vi "Write Priority.vi"(8 "error in (no error)":errorcluster, 10 "Priority":u8, 11 "SearchPriority in":refnum<class "SearchPriority.lvclass">) -> (0 "error out":errorcluster, 3 "SearchPriority out":refnum<class "SearchPriority.lvclass">)   [LabVIEW 2009, in "SearchPriority.lvclass"]
uses:
  SearchPriority.lvclass
  SearchPriority.lvclass/SearchPriority.ctl
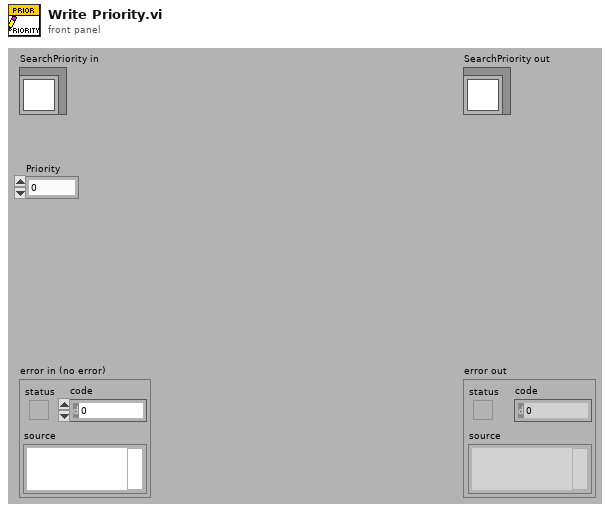
[diagram p1: front panel]
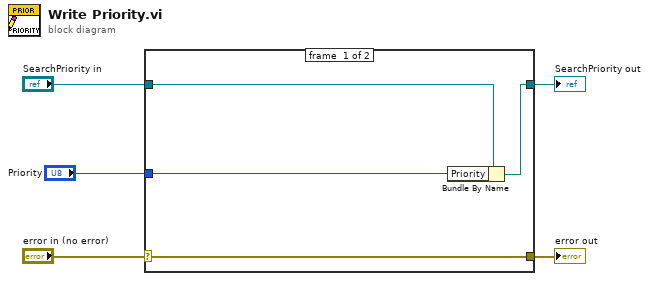
[diagram p0: block diagram]
diagram:
  n1 = case shown="No Error" "error in (no error)" {
    selector: "error in (no error)" -> [w9 w10]
    tunnel: [w9 w10] -> w4
    tunnel: [w7 w11] -> w2
    tunnel: "SearchPriority in" -> [w8 w11]
    tunnel: "Priority" -> [w6 _]
    frame #0 {
      n2 = Bundle By Name(cluster=w8, "Priority"=w6) -> (w7:refnum<class "SearchPriority.lvclass">)
    }
    frame #1 {
    }
  }
  "error out" <- w4
  "SearchPriority out" <- w2
